vi "Simulation - Tank Level Python SW demo3.vi"() -> ()   [LabVIEW 2025]
doc: "This example demonstrates a process simulation for a tank level. The process has added noise, valve deadband, lag, and deadtime. A level controller adjusts the inflow to a tank. An on/off valve serves as a drain that you can click on to operate. This s-valve represents a change in the process loading. You also can switch this VI from automatic control to manual control."
uses:
  <vilib>/addons/control/pid/pid.llb/PID Advanced (DBL).vi
  <vilib>/addons/control/pid/NI_PID_pid.lvlib
panel:
  in  "Tab Control":enum32{"Introduction", "Operation"}(tab)=enum."Operation"
  out "Flow sensor":bool
  in  "HV-101":bool
  out "tank level":dbl(slide) scale=0.0..100.0 scale format="%#.2g"
  out "Valve":bool
  in  "LCV-101":dbl(knob) scale=0.0..100.0
  in  "Auto":bool=TRUE
  out "Process Chart":T1(graph)={"initial PV"=18.934717983735947, "SP(%)"=34.59119496855346, "output"=100.0}
  in  "Setpoint":dbl(slide)=50.0 scale=0.0..100.0
  in  "PID parameters (LIC 101)":T2={"Kc"=10.0, "Ti (min)"=0.05, "Td (min)"=0.0} {"Td (min)" format="%#.6f"; "Ti (min)" format="%#.4f"; "Kc" format="%#.4f"}
  out "flow out":dbl
  out "flow in":dbl
  in  "Stop":bool
  # "Tank Level Control"
  # "Overview: This example demonstrates a process simulation for a tank level.  The process has added noise, valve deadband, lag, and deadtime.  A level controller adjusts the inflow to a tank.  An on/off valve serves as a drain that you can click on to operate.  This s-valve represents a change in the process loading.  You also can switch this VI from automatic control to manual control.\nInstructions:\n1. Run the VI.\n2. Verify the PID controller in closed-loop to track the setpoint.\n3. Change the setpoint to another value and verify the controller tracking the new setpoint.\n4. Apply a disturbance to the system by switching the valve HV 102 (click on the valve symbol). You will see the controller recovering fro the change.\n5. Change PID gains and see if you can improve its performance without going unstable.\n6. Switch to manual mode and see if you can control the level by changing the Valve LVC 101.\n7. Click Stop to stop the VI."
  # "ISA Symbology: The diagram uses the ISA Symbology used for control"
  # "Loop 101"
  # "Level Controller at the control room"
  # "Level Transmitter on the field"
  # "Level Control Valve on the field"
  # "Hand Control Valve on the field"
  # "HV"
  # "102"
  # "LCV"
  # "101"
  # "LIC"
  # "101"
  # "LT"
  # "101"
  # "Slow Leak"
  # "Click to operate"
  # "HV"
  # "102"
  # "LCV"
  # "101"
  # "LIC"
  # "101"
  # "LT"
  # "101"
  # "Manual"
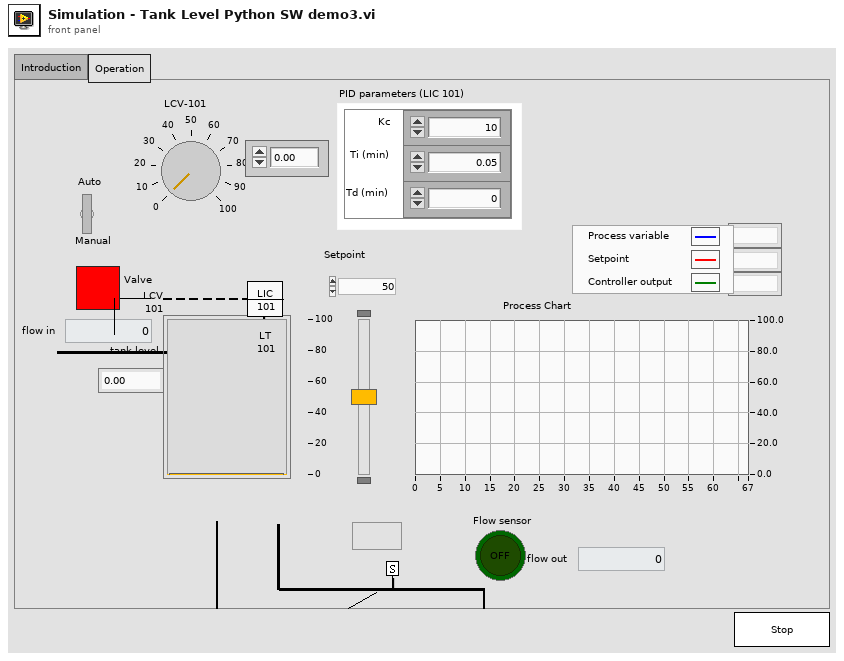
[diagram p1: front panel]
types:
  T1 = cluster{"initial PV":dbl, "SP(%)":dbl, "output":dbl}
  T2 = cluster{"Kc":dbl, "Ti (min)":dbl, "Td (min)":dbl}
  T3 = cluster{"static gain":dbl, "lag (s)":dbl, "deadtime (s)":dbl, "load":dbl, "deadband":dbl, "sensor noise":dbl, "initial PV":dbl, "plant noise":dbl}
  T4 = cluster{"Plant Output":dbl, "Setpoint":dbl, "output":dbl}
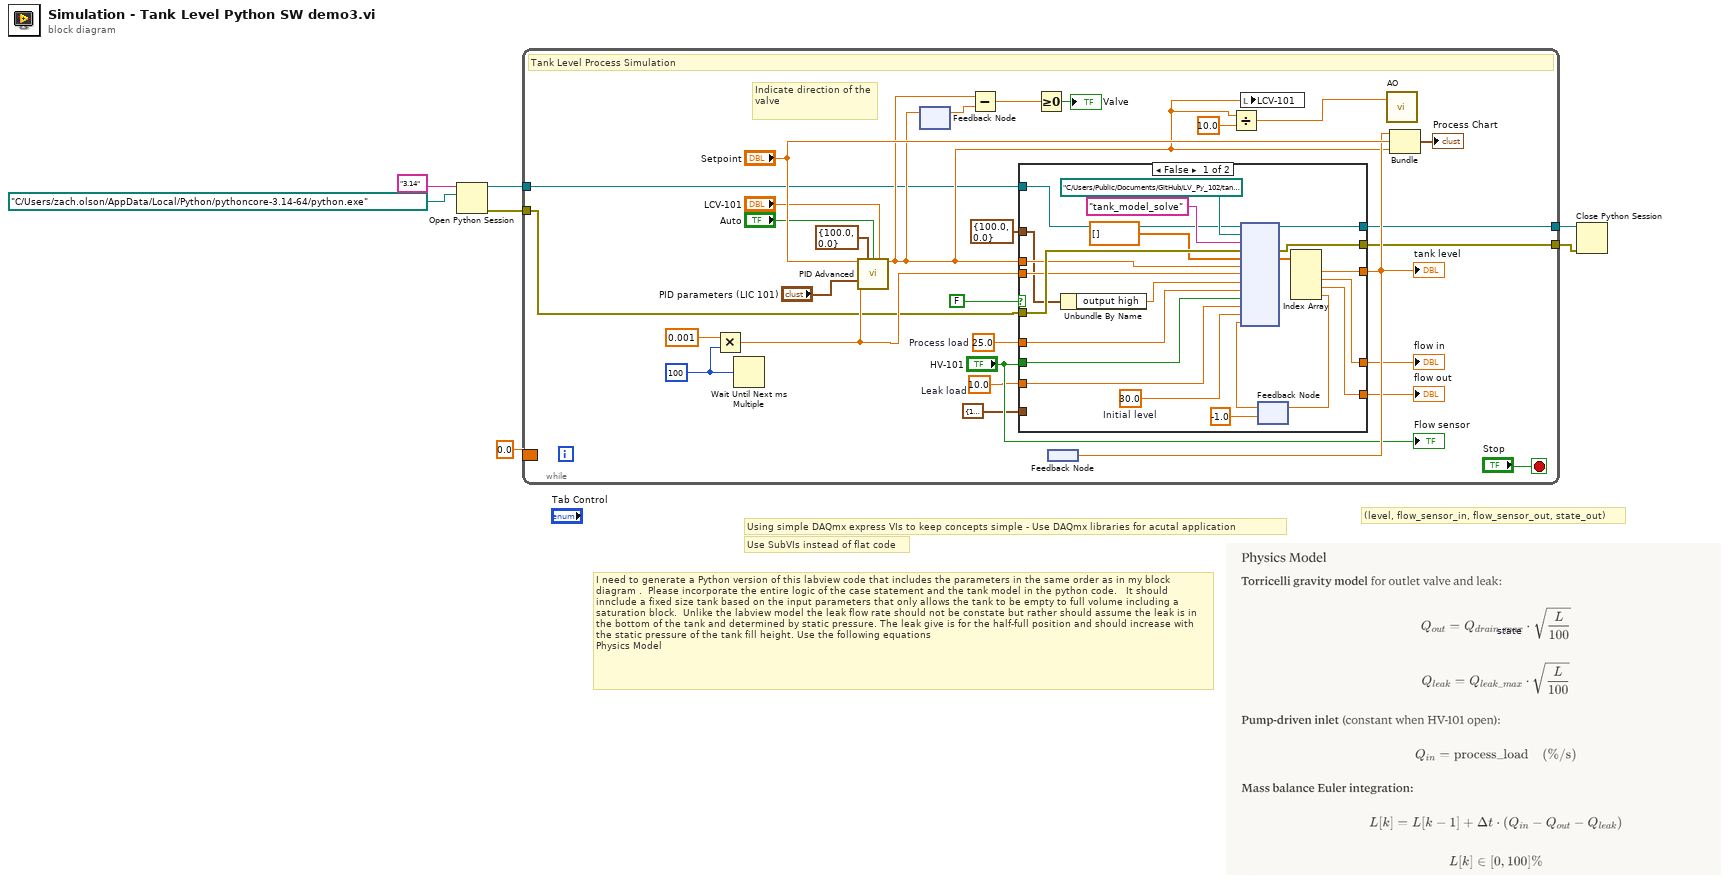
[diagram p0: block diagram]
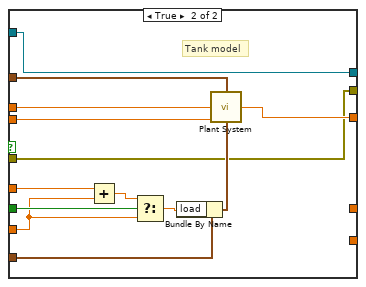
[diagram p2: hidden frame]
diagram:
  # "(level, flow_sensor_in, flow_sensor_out, state_out)"
  # "I need to generate a Python version of this labview code that includes the parameters in the same order as in my block diagram .  Please incorporate the entire logic of the case statement and the tank model in the python code.   It should innclude a fixed size tank based on the input parameters that only allows the tank to be empty to full volume including a saturation block.  Unlike the labview model the leak flow rate should not be constate but rather should assume the leak is in the bottom of the tank and determined by static pressure. The leak give is for the half-full position and should increase with the static pressure of the tank fill height. Use the following equations\nPhysics Model"
  # "Use SubVIs instead of flat code"
  # "Using simple DAQmx express VIs to keep concepts simple - Use DAQmx libraries for acutal application"
  n1 = Open Python Session(python version="3.14" ("Python version"), python path=path "C:/Users/zach.olson/AppData/Local/Python/pythoncore-3.14-64/python.exe" ("Python path")) -> (session out=w4:refnum<k35>, error out=w3:errorcluster)  [unwired: 1 in]
  n2 = while {
    border: 0.0 ("Plant Output") -> [_]
    tunnel: w4 -> [w18]
    tunnel: w3 -> [w17]
    tunnel: [w9] -> w2
    tunnel: [w8] -> w1
    stop <- "Stop" stop-if-true
    w14 = 25.0  # Process load
    w15 = 10.0  # Leak load
    w28 = u32 100
    # "Indicate direction of the valve"
    # "Tank Level Process Simulation"
    n3 = Multiply(x=0.001, y=w28) -> (x*y=w27:dbl)
    n4 = Wait Until Next ms Multiple(millisecond multiple=w28) -> ()  [unwired: 1 out]
    n5 = call-poly <vilib>:"PID Advanced.vi"("setpoint"="Setpoint", "output range"=cluster{"output high":dbl, "output low":dbl} {"output high"=100.0, "output low"=0.0}, "auto? (T)"="Auto", "manual control"="LCV-101", "PID gains"="PID parameters (LIC 101)", "dt (s)"=w27) -> ("output"=w21:dbl)  [unwired: 8 in, 1 out]
    n6 = feedback-in #1(w21) -> ()
    n7 = feedback #1() -> (w25:dbl)  [unwired: 1 in]
    n8 = Subtract(x=w21, y=w25) -> (x-y=w24:dbl)
    n9 = case shown="False" FALSE {
      tunnel: w27 -> [w53 w69]
      tunnel: [w44 w68] -> w26
      tunnel: "HV-101" -> [w50 w66]
      tunnel: w21 -> [w54 w65]
      tunnel: w18 -> [w56 w60]
      tunnel: w17 -> [w55 w59]
      tunnel: w15 -> [w49 w64]
      tunnel: w14 -> [w51 w63]
      tunnel: cluster{"output high":dbl, "output low":dbl} {"output high"=100.0, "output low"=0.0} ("output saturation range") -> [w52 w62]
      tunnel: T3 {"static gain"=1.5, "lag (s)"=18.0, "deadtime (s)"=1.0, "load"=0.0, "deadband"=1.0, "sensor noise"=0.0, "initial PV"=0.0, "plant noise"=5.0} ("process parameters") -> [_ w61]
      tunnel: [w43 _] -> w11
      tunnel: [w42 _] -> w10
      tunnel: [w38 w60] -> w9
      tunnel: [w37 w59] -> w8
      frame False {
        w47 = 30.0  # Initial level
        n10 = Unbundle By Name(w52) -> ("output high"=w48:dbl)
        n11 = feedback #2 "state"(-1.0 ("output low")) -> (w40:dbl)
        n12 = node(w56, path "C:/Users/Public/Documents/GitHub/LV_Py_102/tank.py" ("module path"), "tank_model_solve" ("function name"), w55, dbl[] [], w54, w53, w48, w51, w50, w49, w47, w40) -> (w38:refnum<k35>, w37:errorcluster, w45:dbl[])  [unwired: 8 in, 2 out]
        n13 = Index Array(array=w45) -> (element #1=w44:dbl, element #2=w43:dbl, element #3=w42:dbl, element #4=w41:dbl)  [unwired: 4 in]
        n14 = feedback-in #2(w41) -> ()
      }
      frame True {
        # "Tank model"
        n15 = Add(x=w63, y=w64) -> (x+y=w67:dbl)
        n16 = Select(t=w67, s=w66, f=w64) -> (s? t:f=w71:dbl)
        n17 = Bundle By Name(cluster=w61, "load"=w71) -> (w70:T3)
        n18 = call "Plant System.vi"("output saturation range"=w62, "Plant Input"=w65, "dt (s)"=w69, "process parameters"=w70) -> ("Plant Output"=w68:dbl)  [unwired: 11 in]
      }
    }
    "tank level" <- w26
    "flow out" <- w10
    "flow in" <- w11
    n19 = Greater Or Equal To 0?(x=w24) -> (x >= 0?=→"Valve":bool)
    n20 = feedback-in #3(w26) -> ()
    n21 = feedback #3() -> ()  [unwired: 1 in]
    n22 = Divide(x=w21, y=10.0) -> (x/y=w19:dbl)
    n23 = local write "LCV-101"(w21) -> ()
    n24 = call "AO"("data"=w19) -> ()  [unwired: 17 in, 2 out]
    n25 = Bundle("Plant Output"=w26, "Setpoint"="Setpoint", "output"=w21) -> (→"Process Chart":T4)  [unwired: 1 in]
    "Flow sensor" <- "HV-101"
  }
  n26 = Close Python Session(session in=w2, error in=w1) -> ()  [unwired: 1 out]
